vi "save image.vi"(8 "error in (no error)":errorcluster, 10 "File Path":path, 11 "Thorcam in":refnum<class "Thorcam.lvclass">) -> (0 "error out":errorcluster, 3 "Thorcam out":refnum<class "Thorcam.lvclass">)   [LabVIEW 2012, in "Thorcam.lvclass"]
uses:
  Thorcam.lvclass
  Thorcam.lvclass/Thorcam.ctl
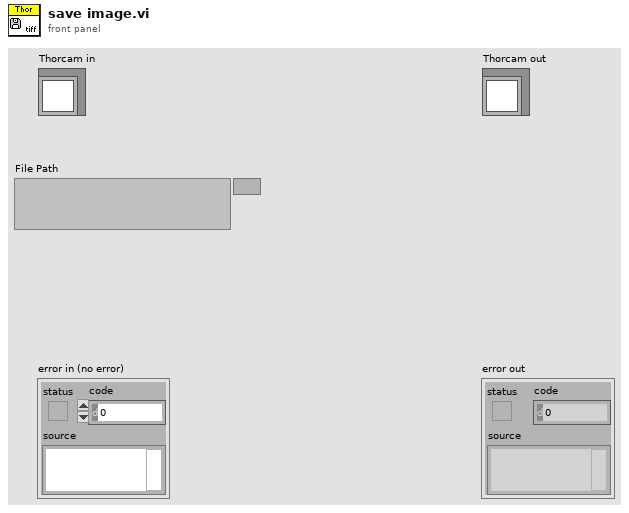
[diagram p1: front panel]
types:
  T1 = cluster{"Rows Per Strip":i32, "Photometric":i32, "Compression Type":i32}
  T2 = typedef "IMAQ Image.ctl" = refnum<image>
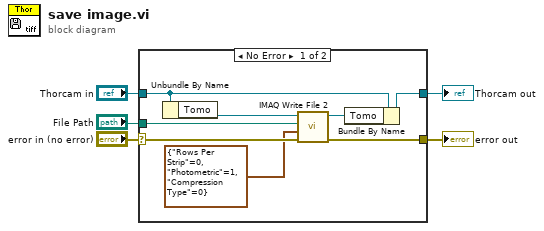
[diagram p0: block diagram]
diagram:
  n1 = case shown="No Error" "error in (no error)" {
    selector: "error in (no error)" -> [w13 w15]
    tunnel: [w12 w15] -> w4
    tunnel: [w7 w14] -> w2
    tunnel: "Thorcam in" -> [w8 w14]
    tunnel: "File Path" -> [w10 _]
    frame No Error {
      n2 = Unbundle By Name(w8) -> ("Tomo"=w9:T2)
      n3 = call-poly "IMAQ Write File 2"("error in (no error)"=w13, "TIFF Options"=T1 {"Rows Per Strip"=0, "Photometric"=1, "Compression Type"=0}, "File Path"=w10, "Image"=w9) -> ("error out"=w12:errorcluster, "Image Out (duplicate)"=w6:T2)  [unwired: 6 in]
      n4 = Bundle By Name(cluster=w8, "Tomo"=w6) -> (w7:refnum<class "Thorcam.lvclass">)
    }
    frame Error {
    }
  }
  "error out" <- w4
  "Thorcam out" <- w2
